vi "Test3.vi"() -> ()   [LabVIEW 2018]
uses:
  6bb7c0b7-d53c-402c-abeb-71b7670bb39b.vi
panel:
  out "주사위 2":i16[](array[numeric])
  out "눈 나온 수 2":i8[](array[numeric])
  in  "눈 나온 수":i8[](array[numeric])
  out "퍼센트":ext[](array[numeric])
  out "주사위":i16[](array[numeric])
  in  "주사위 횟수":i32
  out "~까지 더한거 2":i32
  out "피보나치":i32[](array[numeric])
  in  "숫자형":dbl
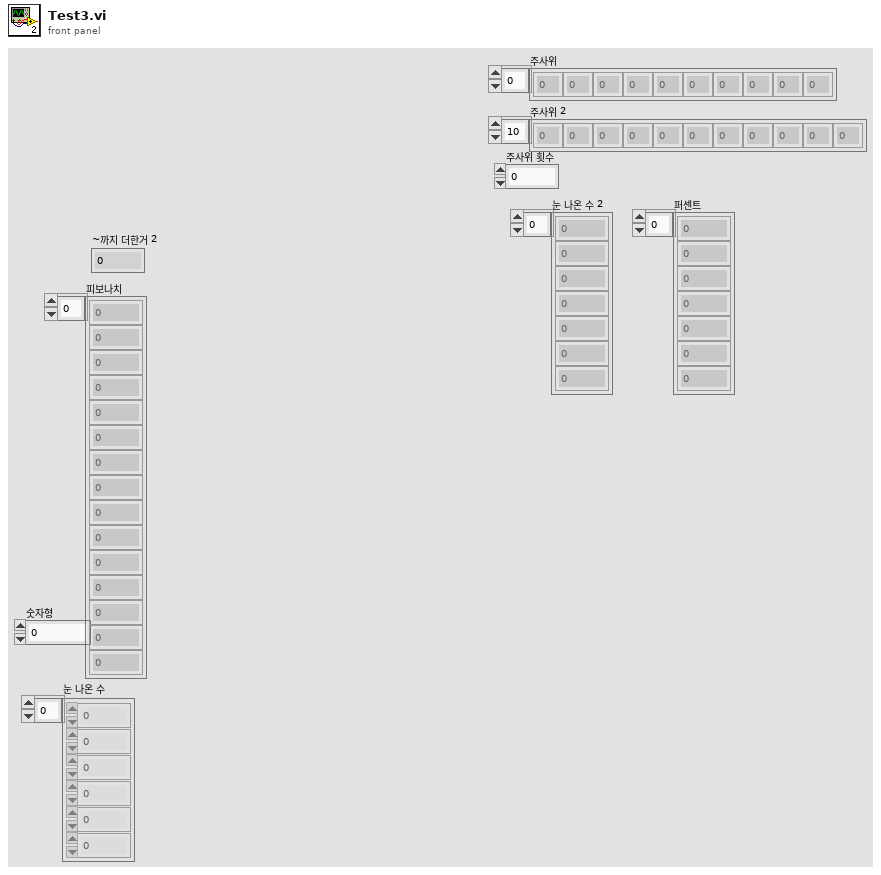
[diagram p1: front panel]
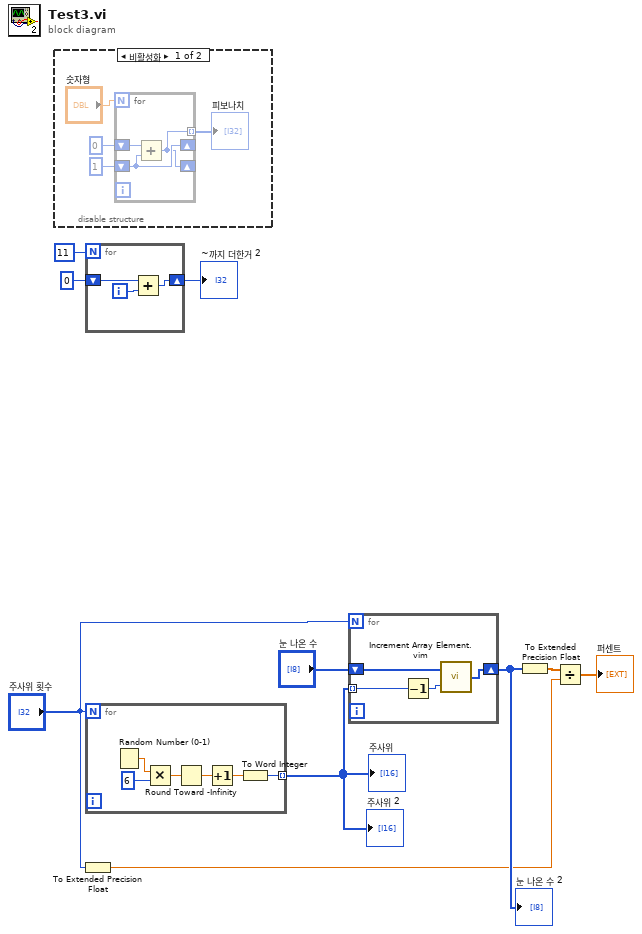
[diagram p0: block diagram]
diagram:
  n1 = disable-structure shown="비활성화" {
    frame Disabled {
      n2 = for {
        N: "숫자형" -> [_]
        shift-right: [w17] -> _
        shift-left: 0 -> [w16]
        shift-right: [w15] -> _
        shift-left: 1 -> [w17]
        tunnel: [w15] -> w11 mode=indexing
        n3 = Add(x=w16, y=w17) -> (x+y=w15:i32)
      }
      "피보나치" <- w11
    }
    frame Enabled {
    }
  }
  n4 = To Extended Precision Float(1:"주사위 횟수") -> (0:w4:ext)
  n5 = for {
    N: 11 -> [_]
    shift-right: [w18] -> w10
    shift-left: 0 -> [w19]
    i -> [w20]
    n6 = Add(x=w19, y=w20) -> (x+y=w18:i32)
  }
  "~까지 더한거 2" <- w10
  n7 = for {
    N: "주사위 횟수" -> [_]
    tunnel: [w26] -> w2 mode=indexing
    n8 = Random Number (0-1)() -> (number: 0 to 1=w21:dbl)
    n9 = Multiply(x=w21, y=6) -> (x*y=w24:dbl)
    n10 = Round Toward -Infinity(1:w24) -> (0:w25:dbl)
    n11 = Increment(x=w25) -> (x+1=w23:dbl)
    n12 = To Word Integer(number=w23) -> (16bit integer=w26:i16)
  }
  "주사위" <- w2
  "주사위 2" <- w2
  n13 = for {
    N: "주사위 횟수" -> [_]
    shift-right: [w27] -> w6
    shift-left: "눈 나온 수" -> [w29]
    tunnel: w2 -> [w30] mode=indexing
    n14 = Decrement(x=w30) -> (x-1=w28:i16)
    n15 = call "Increment Array Element.vim"("index"=w28, "array in"=w29) -> ("array out"=w27:i8[])
  }
  "눈 나온 수 2" <- w6
  n16 = To Extended Precision Float(1:w6) -> (0:w3:ext[])
  n17 = Divide(x=w3, y=w4) -> (x/y=→"퍼센트":ext[])
